vi "CAN test.vi"() -> ()   [LabVIEW 2017]
uses:
  NI CAN VIS/New folder/CAN_OPERATION _TYPEDEF.ctl
  94919273-0e9c-4002-9f15-977baf55949d.vi
  3b1876b6-6c64-4131-aa3f-14275e53b31f.vi
  CAN Specific to this project/Serial Number Write.ctl
  CAN Specific to this project/CAN CMD-RES PARA.ctl
  CAN Specific to this project/CAN Specific Cluster.ctl
  Controls/Indicator Status Large.ctl
  Controls/App Control/Inspection Control.ctl
  <vilib>/Utility/miscctls.llb/LVRowAndColumnTypeDef.ctl
  <vilib>/Utility/miscctls.llb/LVPositionTypeDef.ctl
  Controls/App Control/PGS Cluster Data.ctl
  Controls/App Control/PGS Control.ctl
panel:
  in  "Main Screen Cluster input 2":T1
  in  "Multicolumn Listbox":i32(listbox)
  out "Actual CAN Array 4":string[][](array[string])
  out "Error out 4":errorcluster {"code" format="%.0x"}
  in  "Error in 3":errorcluster {"code" format="%.0x"}
  in  "Boolean 2":bool
  out "Actual CAN Array 3":string[][](array[string])
  out "Actual CAN Array 2":string[][](array[string])
  in  "WRITE CMD":u8[](array[numeric])=[0, 0, 0, 0, 0, 0, 0, 0, 241, 16, 0, 0, 0, 0, 0, 0] format="%.0x"
  out "Actual CAN Array":string[][](array[string])
  in  "Boolean":bool
  out "Error out 2":errorcluster {"code" format="%.0x"}
  in  "Error in 2":errorcluster {"code" format="%.0x"}
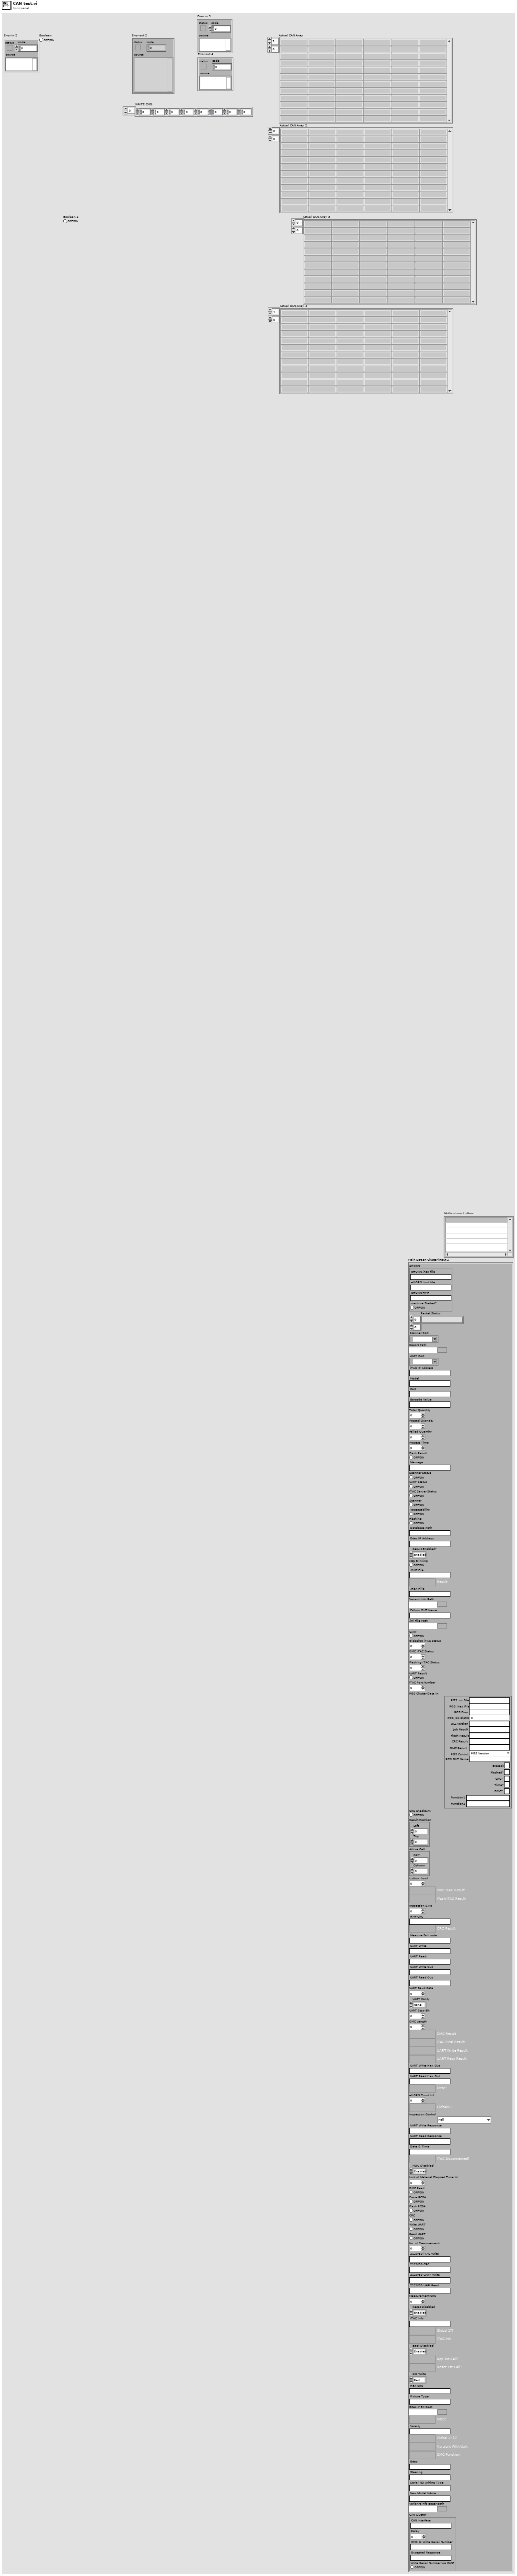
[diagram p1: front panel]
types:
  T1 = typedef "Msg Cluster Data.ctl" = cluster{"eHORN":T2, "Packet Status":string[][], "Scanner Port":refnum<visa-resource-name>, "Report Path":path, "UART Port":refnum<visa-resource-name>, "iTAC IP Address":string, "Model":string, "Part":string, "Barcode Value":string, "Total Quantity":u64, "Passed Quantity":u64, "Failed Quantity":u64, "Process Time":u64, "Flash Result":bool, "Message":string, "Scanner Status":T3, "UART Status":T3, "iTAC Server Status":T3, "Scanner":T3, "Traceasability":T3, "Flashing":T3, "Database Path":string, "Ertec IP Address":string, "Result Enabled?":enum8{"Enabled", "Disabled", "Disabled and Grayed Out"}, "Msg Blinking":bool, ".HMF File":string, "Result":T4, ".HEX Fille":string, "Variant Info Path":path, "E-Horn DUT Name":string, ".ini File Path":path, "UART":T3, "Global00 iTAC Status":i64, "DMC iTAC Status":i64, "Flashing iTAC Status":i64, "UART Result":T3, "iTAC Port Number":u16, "PGS Cluster Data In":T5, "CRC Checksum":T3, "Result Position":T7, "Active Cell":T8, "Listbox (row)":i32, "DMC iTAC Result":T4, "Flash iTAC Result":T4, "Inspection S.No":u8, "HMF CRC":string, "CRC Result":T4, "Measure Fail code":string, "UART Write":string, "UART Read":string, "UART Write Out":string, "UART Read Out":string, "UART Baud Rate":u32, "UART Parity":enum16{"None", "Odd", "Even", "Mark", "Space"}, "UART Stop Bit":u16, "DMC Length":u8, "DMC Result":T4, "iTAC Final Result":T4, "UART Write Result":T4, "UART Read Result":T4, "UART Write Hex Out":string, "UART Read Hex Out":string, "Error?":T4, "eHORN Count (s)":u64, "Global01?":T4, "Inspection Control":T9, "UART Write Response":string, "UART Read Response":string, "Date & Time":string, "iTAC Disconnected?":T4, "MDC Disabled":enum8{"Enabled", "Disabled", "Disabled and Grayed Out"}, "Lock of Material Elapsed Time (s)":u8, "DMC Read":bool, "Erase PCBA":bool, "Flash PCBA":bool, "CRC":bool, "Write UART":bool, "Read UART":bool, "No. of Measurements":u8, "2120/30 iTAC Write":string, "2120/30 CRC":string, "2120/30 UART Write ":string, "2120/30 UARt Read":string, "Measurement CRC":u8, "Reset Disabled":enum8{"Enabled", "Disabled", "Disabled and Grayed Out"}, "iTAC Info":string, "Global 17?":T4, "iTAC Init":T4, "Back Disabled":enum8{"Enabled", "Disabled", "Disabled and Grayed Out"}, "App 1st Call?":T4, "Reset 1st Call?":T4, "DO Write":T10, "HEX CRC":string, "Fixture Type":string, "Ertec .HEX Root":path, "MDC?":T4, "Vareity":string, "Global 17 (2)":T4, "Varaiant With Uart":T4, "DMC Function":T4, "Ertec":string, "Steering":string, "Serial NO writing Type":string, "New Model NAme":string, "Varianrt info Baser path":path, "CAN Cluster":cluster{"CAN Interface":string, "Delay":dbl, "CMD to Write Serial Number":string, "Excepted Response":string, "Write Serial Number via CAN?":bool}}
  T2 = typedef "User.ctl" = cluster{"eHORN .hex file":string, "eHORN .hmf file":string, "eHORN HMF":string, "machine Started?":bool}
  T3 = typedef "Indicator Status Small.ctl" = bool
  T4 = typedef "Indicator Status Large.ctl" = bool
  T5 = typedef "PGS Cluster Data.ctl" = cluster{"PGS .ini File":string, "PGS .hex File":string, "PGS Error":string, "PGS Job SlotID":u32, "DLL Version":string, "Job Result":string, "Flash Result":string, "CRC Result":string, "PGS Control":T6, "PGS DUT Name":string, "Erased?":bool, "Flashed?":bool, "CRC?":bool, "Time?":bool, "DMC Result":string, "DMC?":bool, "Function1":string, "Function2":string}
  T6 = typedef "PGS Control.ctl" = enum16{"PGS Version", "PGS Setup", "PGS Job Open", "Open Delay", "Ertec HW Status", "Ertec HW Status Time Delay", "PGS Erase", "Erase Delay", "Erase Ready", "PGS Job Start", "Start Delay", "PGS Flash Result", "PGS Time Delay", "Write Delay", "PGS Checksum", "PGS CRC Delay", "Delay", "DMC Function 1", "Function 1 Delay", "DMC Function 2", "Function 2 Delay", "PGS Job Result", "PGS Job Result Delay", "PGS Job Close", "PGS Exit", "PGS Error"}
  T7 = typedef "LVPositionTypeDef.ctl" = cluster{"Left":i32, "Top":i32}
  T8 = typedef "LVRowAndColumnTypeDef.ctl" = cluster{"Row":i32, "Column":i32}
  T9 = typedef "Inspection Control.ctl" = enum16{"Poll", "Global Initialize", "Dynamic Launch", "Initialize", "Identify Fixture", "iTAC Status", "Scanner Status", "UART Staus", "Global 20", "Hardware Status", "Scan Barcode", "Process Precheck", "DMC iTAC Traceability Msg", "DMC iTAC Traceability", "Global 00", "Ertec Flash Msg", "Ertec Erase", "Ertec Flash", "Checksum Calculation Msg", "Checksum Precheck", "Checksum Calculation", "Checksum Verification Msg", "Checksum Verification", "UART Msg", "UART Write Cmd", "UART Write Result", "UART Write Response", "UART Read Delay", "UART Read Cmd", "UART Read Result", "UART Read Response", "Steering Switch DMC", "iTAC Traceability Msg", "Result iTAC Traceability", "Result", "Save Result", "DUT Remove", "Test Initialize", "Open UART", "Reset", "Rejection Bin", "LID Sensor", "VCC 12V/24V Relay", "Global 01", "Machine Error", "Global 17", "MDC Access", "Process Reset", "Rejection Sensor", "Serial Number Write Via CAN", "Exit"}
  T10 = typedef "Digital Input Control.ctl" = enum16{"Red", "Amber", "Green", "Buzzer", "VCC 24V DC", "VCC 12V DC", "Spare1", "Spare2", "Spare3", "Spare4", "Spare5", "Spare6", "Spare7", "Spare8", "Spare9", "Spare10"}
  T11 = typedef "CAN_OPERATION _TYPEDEF.ctl" = string
  T12 = typedef "CAN Specific Cluster.ctl" = cluster{"EOL Sesion Entry P":T13, "ECU Test Entry":T13, "Write Serial Number F1":T13, "Write Serial Number F2":T13, "Write Serial Number F3":T13, "Error Message":string, "Result":cluster{"Default mess":bool, "EOL Session":bool, "ECU Test ENtry":bool, "CAN WR F1":bool, "CAN WR F2":bool, "CAN WR F3":bool, "CAN R F1":bool, "CAN R F2":bool, "CAN R F3":bool}, "Inspection Control":dbl, "Packet Status":string[][]}
  T13 = typedef "CAN CMD-RES PARA.ctl" = cluster{"CMD ":u8[], "Response":u8[], "DLC":i32, "CMD AR ID":i32, "RES AR ID":i32}
  T14 = typedef "Serial Number Write.ctl" = enum16{"Error", "Serial NO R F3", "Serial NO R F2", "Serial NO R F1", "Serial NO Wr F3", "Serial NO Wr F2", "Serial NO Wr F1", "Verify ECU Test Entry ", "ECU Test Entry", "Verify EOl Session Entry", "Enter EOl Session", "Read Default Mess", "Exit", "INI"}
  T15 = typedef "Serial Number Write.ctl" = enum16{"Error", "Serial Number Read", "Serial Number Write", "Verify ECU Test Entry ", "ECU Test Entry", "Verify EOl Session Entry", "Enter EOl Session", "Read Default Mess", "Exit", "INI"}
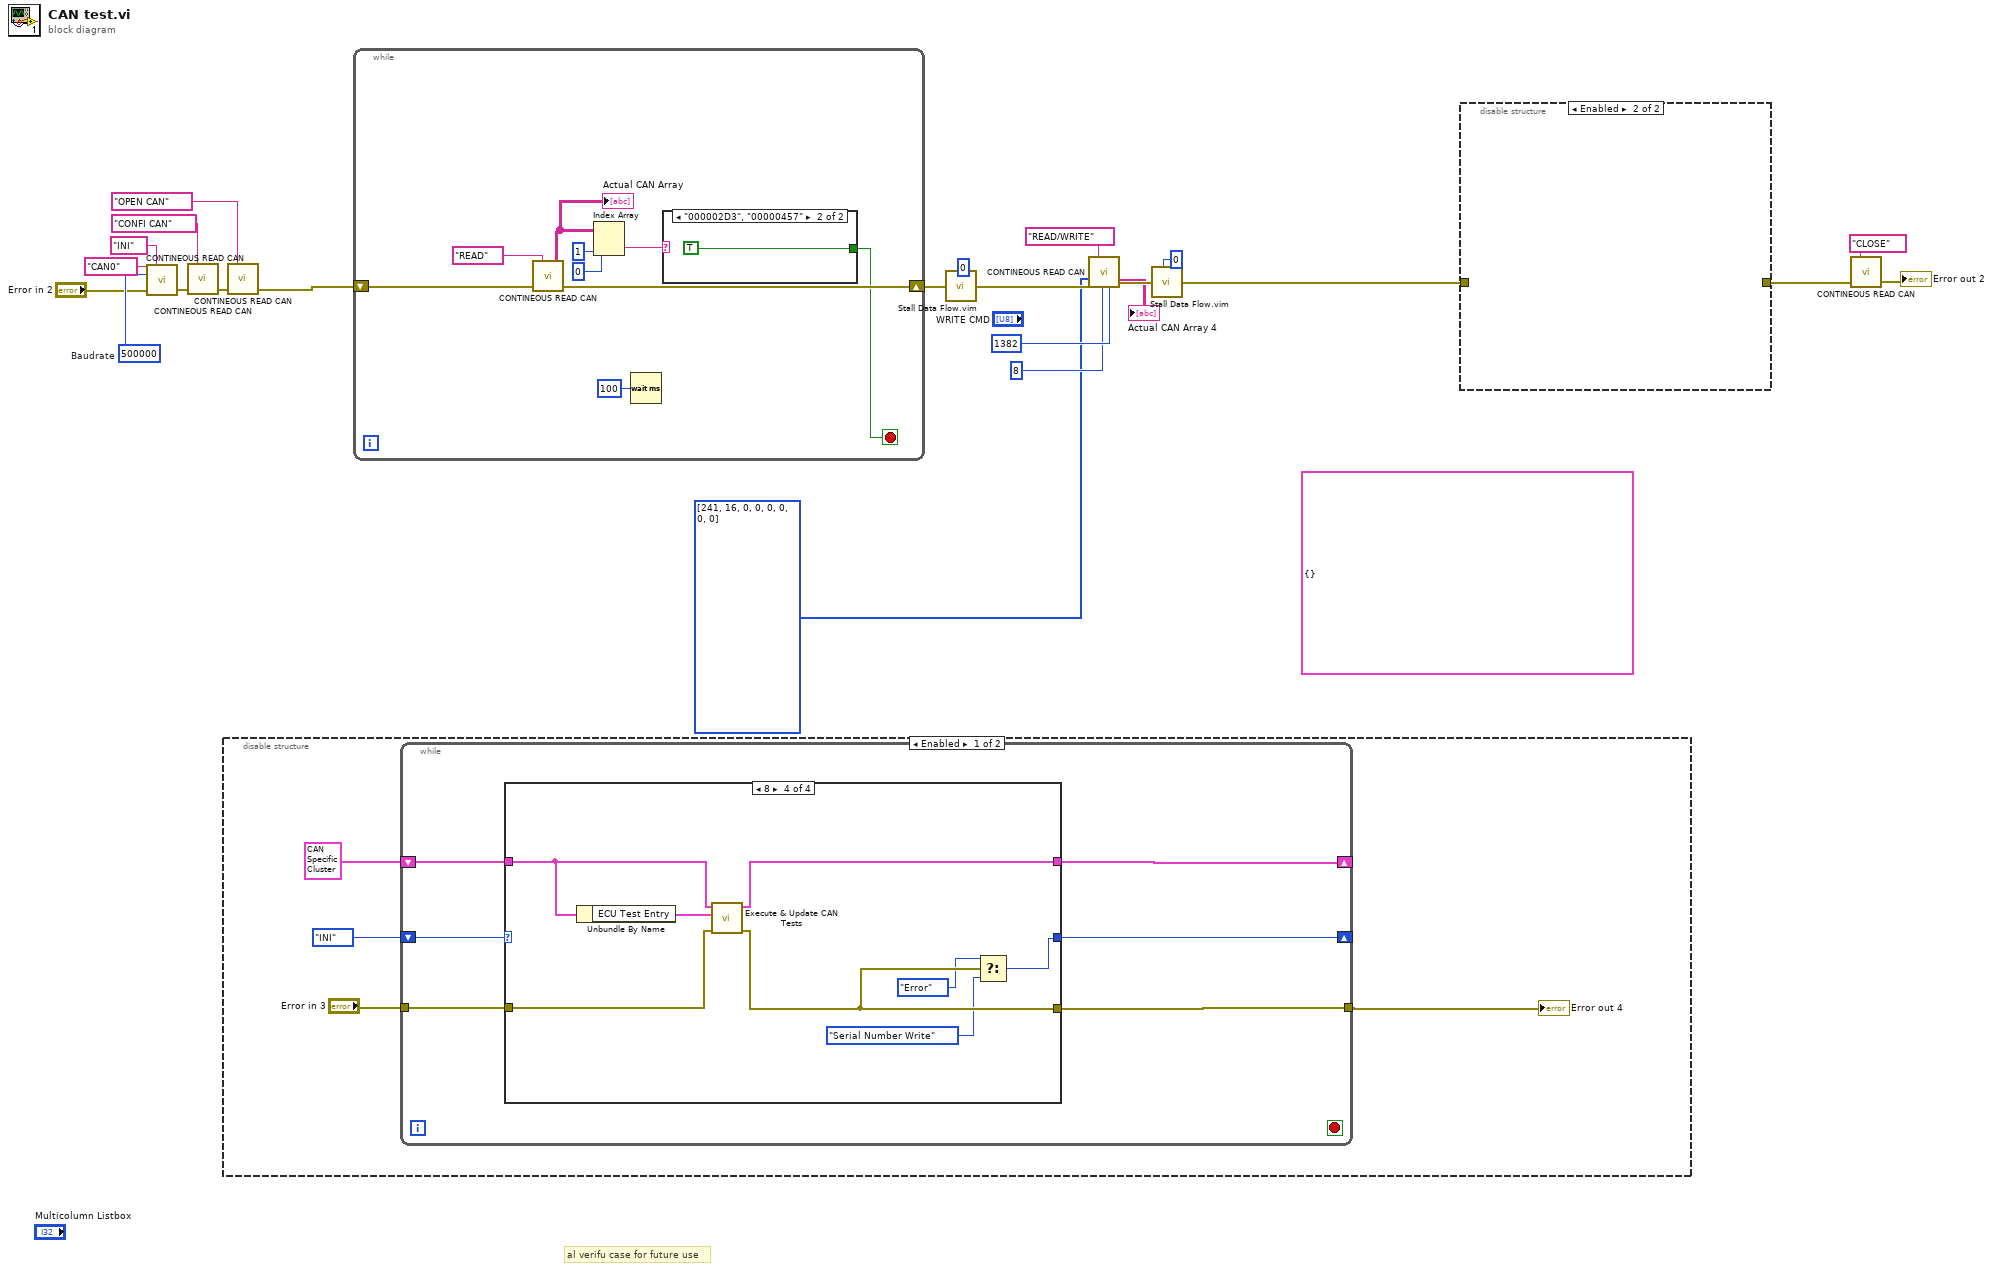
[diagram p0: block diagram]
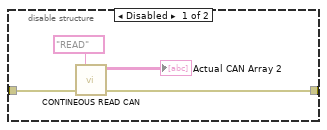
[diagram p2: hidden frame]
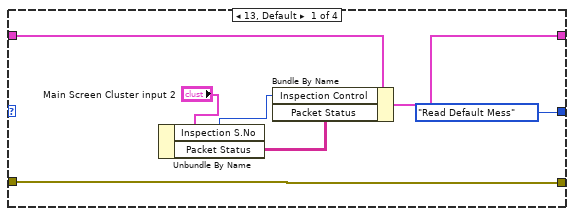
[diagram p3: hidden frame]
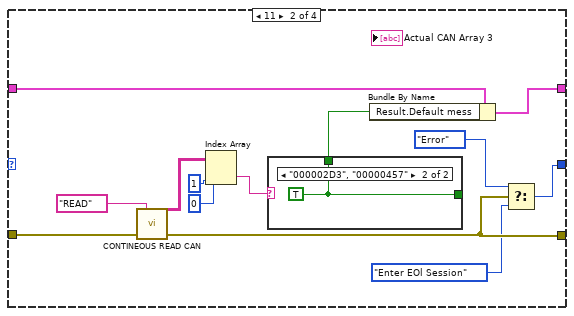
[diagram p4: hidden frame]
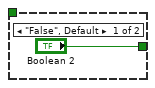
[diagram p5: hidden frame]
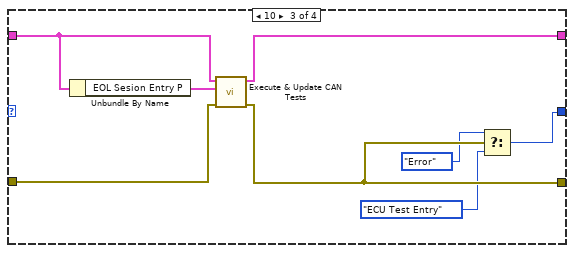
[diagram p6: hidden frame]
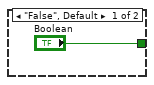
[diagram p8: hidden frame]
diagram:
  (unwired) cluster{} {}
  w18 = u32 500000  # Baudrate
  # "al verifu case for future use"
  n1 = call "CONTINEOUS READ CAN.vi"("interface"="CAN0", "Baudrate"=w18, "Error in 2"="Error in 2", "CAN OPERATION"=T11 "INI") -> ("Error out 2"=w20:errorcluster)  [unwired: 17 in, 6 out]
  n2 = call "CONTINEOUS READ CAN.vi"("Error in 2"=w20, "CAN OPERATION"=T11 "CONFI CAN") -> ("Error out 2"=w19:errorcluster)  [unwired: 19 in, 6 out]
  n3 = disable-structure shown="Enabled" {
    frame Enabled {
      n4 = while {
        shift-right: [w32] -> _
        shift-left: Serial_Number_Write."INI" -> [w33]
        tunnel: "Error in 3" -> [w31]
        tunnel: [w30] -> w25
        shift-right: [w29] -> _
        shift-left: T12 {"EOL Sesion Entry P"={"CMD "=[241, 16, 0, 0, 0, 0, 0, 0], "Response"=[241, 16, 0, 0, 0, 0, 0, 0], "DLC"=0, "CMD AR ID"=0, "RES AR ID"=0}, "ECU Test Entry"={"CMD "=[241, 16, 0, 0, 0, 0, 0, 0], "Response"=[241, 16, 0, 0, 0, 0, 0, 0], "DLC"=0, "CMD AR ID"=0, "RES AR ID"=0}, "Write Serial Number F1"={"CMD "=[241, 16, 0, 0, 0, 0, 0, 0], "Response"=[241, 16, 0, 0, 0, 0, 0, 0], "DLC"=0, "CMD AR ID"=0, "RES AR ID"=0}, "Write Serial Number F2"={"CMD "=[241, 16, 0, 0, 0, 0, 0, 0], "Response"=[241, 16, 0, 0, 0, 0, 0, 0], "DLC"=0, "CMD AR ID"=0, "RES AR ID"=0}, "Write Serial Number F3"={"CMD "=[241, 16, 0, 0, 0, 0, 0, 0], "Response"=[241, 16, 0, 0, 0, 0, 0, 0], "DLC"=0, "CMD AR ID"=0, "RES AR ID"=0}, "Error Message"="", "Result"={"Default mess"=FALSE, "EOL Session"=FALSE, "ECU Test ENtry"=FALSE, "CAN WR F1"=FALSE, "CAN WR F2"=FALSE, "CAN WR F3"=FALSE, "CAN R F1"=FALSE, "CAN R F2"=FALSE, "CAN R F3"=FALSE}, "Inspection Control"=0.0, "Packet Status"=[]} -> [w28]
        stop <- _ stop-if-true
        n5 = case shown="8" w33 {
          tunnel: [Serial_Number_Write."Read Default Mess" w48 w63 w71] -> w32
          tunnel: w31 -> [w39 w47 w61 w69]
          tunnel: [w39 w43 w58 w66] -> w30
          tunnel: [w37 w45 w62 w70] -> w29
          tunnel: w28 -> [w38 w46 w60 w68]
          frame 13, Default {
            n6 = Unbundle By Name("Main Screen Cluster input 2") -> ("Inspection S.No"=w35:u8, "Packet Status"=w34:string[][])
            n7 = Bundle By Name(cluster=w38, "Inspection Control"=w35, "Packet Status"=w34) -> (w37:T12)
          }
          frame 11 {
            n8 = call "CONTINEOUS READ CAN.vi"("Error in 2"=w47, "CAN OPERATION"=T11 "READ") -> ("Actual CAN Array"=w49:string[][], "Error out 2"=w43:errorcluster)  [unwired: 19 in, 5 out]
            n9 = Index Array(array=w49, index (row)=0 ("disabled index (row)"), index (col)=1 ("disabled index (col)")) -> (element=w52:string)
            n10 = case shown="\"000002D3\", \"00000457\"" w52 {
              tunnel: ["Boolean 2" w55] -> _
              tunnel: [_ w55] -> w44
              frame "False", Default {
              }
              frame "000002D3", "00000457" {
                w55 = TRUE
              }
            }
            n11 = Bundle By Name(cluster=w46, "Result.Default mess"=w44) -> (w45:T12)
            n12 = Select(t=Serial_Number_Write."Error", s=w43, f=Serial_Number_Write."Enter EOl Session") -> (s? t:f=w48:T14)
          }
          frame 10 {
            n13 = Unbundle By Name(w60) -> ("EOL Sesion Entry P"=w59:T13)
            n14 = call "Execute & Update CAN Tests.vi"("Error in 3"=w61, "EOL Sesion Entry P"=w59, "input cluster"=w60) -> ("Error in 4"=w58:errorcluster, "input cluster 2"=w62:T12)  [unwired: 7 in]
            n15 = Select(t=Serial_Number_Write."Error", s=w58, f=Serial_Number_Write."ECU Test Entry") -> (s? t:f=w63:T14)
          }
          frame 8 {
            n16 = Unbundle By Name(w68) -> ("ECU Test Entry"=w67:T13)
            n17 = call "Execute & Update CAN Tests.vi"("Error in 3"=w69, "EOL Sesion Entry P"=w67, "input cluster"=w68) -> ("Error in 4"=w66:errorcluster, "input cluster 2"=w70:T12)  [unwired: 7 in]
            n18 = Select(t=Serial_Number_Write."Error", s=w66, f=Serial_Number_Write."Serial Number Write") -> (s? t:f=w71:u16)
          }
        }
      }
      "Error out 4" <- w25
    }
    frame Disabled {
    }
  }
  n19 = call "CONTINEOUS READ CAN.vi"("Error in 2"=w19, "CAN OPERATION"=T11 "OPEN CAN") -> ("Error out 2"=w17:errorcluster)  [unwired: 19 in, 6 out]
  n20 = while {
    shift-right: [w75] -> w16
    shift-left: w17 -> [w80]
    stop <- w73 stop-if-true
    n21 = call "CONTINEOUS READ CAN.vi"("Error in 2"=w80, "CAN OPERATION"=T11 "READ") -> ("Actual CAN Array"=w79:string[][], "Error out 2"=w75:errorcluster)  [unwired: 19 in, 5 out]
    "Actual CAN Array" <- w79
    n22 = Index Array(array=w79, index (row)=0 ("disabled index (row)"), index (col)=1 ("disabled index (col)")) -> (element=w76:string)
    n23 = Wait (ms)(milliseconds to wait=u32 100) -> ()  [unwired: 1 out]
    n24 = case shown="\"000002D3\", \"00000457\"" w76 {
      tunnel: ["Boolean" TRUE] -> w73
      frame "False", Default {
      }
      frame "000002D3", "00000457" {
      }
    }
  }
  n25 = call "Stall Data Flow.vim"("value in"=w16, "milliseconds to wait"=u32 0) -> ("value out"=w4:errorcluster)  [unwired: 1 out]
  n26 = call "CONTINEOUS READ CAN.vi"("WRITE CMD"=u8[] [241, 16, 0, 0, 0, 0, 0, 0], "Error in 2"=w4, "CAN OPERATION"=T11 "READ/WRITE", "WRITE AR ID"=u32 1382, "DataLength"=u32 8) -> ("Actual CAN Array"=→"Actual CAN Array 4":string[][], "Error out 2"=w9:errorcluster)  [unwired: 16 in, 5 out]
  n27 = call "Stall Data Flow.vim"("value in"=w9, "milliseconds to wait"=u32 0) -> ("value out"=w7:errorcluster)  [unwired: 1 out]
  n28 = disable-structure shown="Enabled" {
    disable-tunnel: [w86 _] -> w8
    disable-tunnel: w7 -> [w85 _]
    frame Disabled {
      n29 = call "CONTINEOUS READ CAN.vi"("Error in 2"=w85, "CAN OPERATION"=T11 "READ") -> ("Actual CAN Array"=→"Actual CAN Array 2":string[][], "Error out 2"=w86:errorcluster)  [unwired: 19 in, 5 out]
    }
    frame Enabled {
    }
  }
  n30 = call "CONTINEOUS READ CAN.vi"("Error in 2"=w8, "CAN OPERATION"=T11 "CLOSE") -> ("Error out 2"=→"Error out 2":errorcluster)  [unwired: 19 in, 6 out]
